vi "MGI Read Anything.vi"(5 "Read/Write Options (Version 1.x)":T1={"TS Fmt"="%04Y%02m%02d %02H%02M%S%25u", "Int Fmt"="%d", "Delimiter"=""}, 6 "Use Supplied (F: Use Default)":bool, 7 "Type of Anything":variant, 8 "Error In":errorcluster, 9 "Section Name (Name of \"Type of Anything\")":string, 10 "Format String (%#_13g)":string="%#_13g", 11 "Path (dialog)":path) -> (0 "Error Out":errorcluster, 1 "Found?":bool, 2 "Read Failures":string, 3 "Anything":variant)   [LabVIEW 2018]
doc: "This VI is designed to read data from a file written by <B>Write Anything.vi</B>. If the data type definition has changed since it was written to file, this VI will still read and fill out any elements of the cluster that have the same name. Any elements for which it cannot find a name match in the file will be supplied with their datatype's default value if Use Supplied is false. If \"Use Supplied\" is true, any elements whose name is not found in the file will use the data in the corresponding field of Type of Anything.\n\"Read/Write Options (Version 1.x)\" is used if the file at the specified Path was written with MGI Write Anything version 1.x. If the file was written with MGI Write Anything Version 2.0 or later, than the \"Read/Write Options (Version 1.x)\" input is ignored since these parameters are stored in the data file itself.\nAuthored by Robert C. Mortensen\nsupport@mooregoodideas.com\nwww.mooregoodideas.com\n\nCopyright (c) 2010, Moore Good Ideas, Inc.\n\nAll rights reserved.\n\nRedistribution and use in source and binary forms, with or without modification, are permitted provided that the following conditions are met:\n\n * Redistributions of source code must retain the above copyright notice, this list of conditions and the following disclaimer.\n * Redistributions in binary form must reproduce the above copyright notice, this list of conditions and the following disclaimer in the documentation and/or other materials provided with the distribution.\n * Neither the name of Moore Good Ideas, Inc. nor the names of its contributors may be used to endorse or promote products derived from this software without specific prior written permission.\n\nTHIS SOFTWARE IS PROVIDED BY THE COPYRIGHT HOLDERS AND CONTRIBUTORS \"AS IS\" AND ANY EXPRESS OR IMPLIED WARRANTIES, INCLUDING, BUT NOT LIMITED TO, THE IMPLIED WARRANTIES OF MERCHANTABILITY AND FITNESS FOR A PARTICULAR PURPOSE ARE DISCLAIMED. IN NO EVENT SHALL THE COPYRIGHT OWNER OR CONTRIBUTORS BE LIABLE FOR ANY DIRECT, INDIRECT, INCIDENTAL, SPECIAL, EXEMPLARY, OR CONSEQUENTIAL DAMAGES (INCLUDING, BUT NOT LIMITED TO, PROCUREMENT OF SUBSTITUTE GOODS OR SERVICES; LOSS OF USE, DATA, OR PROFITS; OR BUSINESS INTERRUPTION) HOWEVER CAUSED AND ON ANY THEORY OF LIABILITY, WHETHER IN CONTRACT, STRICT LIABILITY, OR TORT (INCLUDING NEGLIGENCE OR OTHERWISE) ARISING IN ANY WAY OUT OF THE USE OF THIS SOFTWARE, EVEN IF ADVISED OF THE POSSIBILITY OF SUCH DAMAGE."
uses:
  MGI RWA Options Cluster.ctl
  VariantType.lvlib
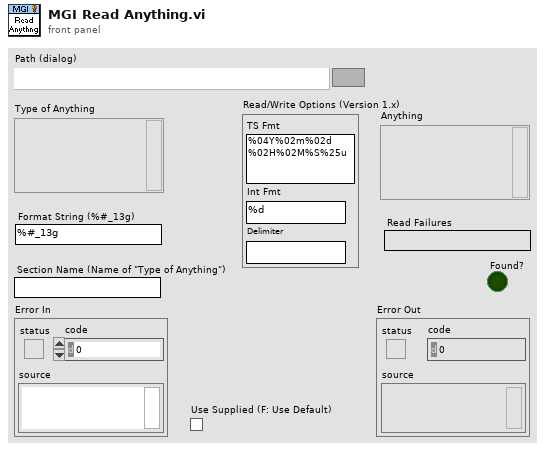
[diagram p1: front panel]
types:
  T1 = typedef "MGI RWA Options Cluster.ctl" = cluster{"TS Fmt":string, "Int Fmt":string, "Delimiter":string}
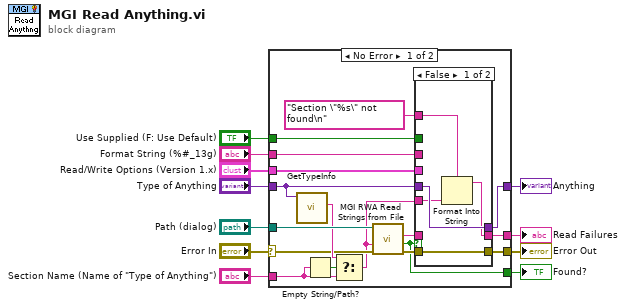
[diagram p0: block diagram]
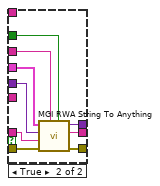
[diagram p2: hidden frame]
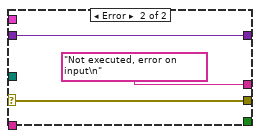
[diagram p3: hidden frame]
diagram:
  n1 = case shown="No Error" "Error In" {
    selector: "Error In" -> [w19 w45]
    tunnel: [w28 w45] -> w11
    tunnel: [w27 w44] -> w10
    tunnel: [w17 _] -> w9
    tunnel: "Path (dialog)" -> [w25 _]
    tunnel: "Section Name (Name of \"Type of Anything\")" -> [w23 _]
    tunnel: "Type of Anything" -> [w21 w44]
    tunnel: "Read/Write Options (Version 1.x)" -> [w20 _]
    tunnel: "Format String (%#_13g)" -> [w16 _]
    tunnel: "Use Supplied (F: Use Default)" -> [w15 _]
    tunnel: [w14 "Not executed, error on input\n"] -> w1
    frame No Error {
      n2 = call "GetTypeInfo.vi"("Variant"=w21) -> ("Name"=w22:string)  [unwired: 6 in, 4 out]
      n3 = Empty String/Path?(string/path=w23) -> (empty?=w24:bool)
      n4 = Select(t=w22, s=w24, f=w23) -> (s? t:f=w13:string)
      n5 = call "MGI RWA Read Strings from File.vi"("Error In"=w19, "Section Name"=w13, "Path"=w25) -> ("Error Out"=w26:errorcluster, "Found?"=w17:bool, "String"=w18:string)  [unwired: 6 in]
      n6 = case shown="False" w17 {
        tunnel: [w32 w42] -> w28
        tunnel: [w33 w41] -> w27
        tunnel: w21 -> [w33 w39]
        tunnel: w26 -> [w32 w40]
        tunnel: w20 -> [_ w38]
        tunnel: w18 -> [_ w37]
        tunnel: w16 -> [_ w35]
        tunnel: w15 -> [_ w36]
        tunnel: [w30 w34] -> w14
        tunnel: w13 -> [w31 _]
        tunnel: "Section \"%s\" not found\n" ("format string") -> [w29 _]
        frame False {
          n7 = Format Into String(format string=w29, w31) -> (resulting string=w30:string)  [unwired: 2 in, 1 out]
        }
        frame True {
          n8 = call "MGI RWA String To Anything.vi"("Use Supplied"=w36, "Format String (%#_13g)"=w35, "Error In"=w40, "String"=w37, "Type of Anything"=w39, "Read/Write Options"=w38) -> ("Error Out"=w42:errorcluster, "Read Failures"=w34:string, "Variant"=w41:variant)  [unwired: 3 in]
        }
      }
    }
    frame Error {
    }
  }
  "Error Out" <- w11
  "Anything" <- w10
  "Found?" <- w9
  "Read Failures" <- w1
